vi "Filter Only Tomestones.vi"(8 "Error In":errorcluster, 11 "VI Bookmarks":T1[](array[typedef])) -> (0 "Error Out":errorcluster, 3 "Graves":T1[](array[typedef]))   [LabVIEW 2017, in "Graveyard.lvlib"]
doc: "Filters out all bookmarks that are NOT graves"
uses:
  Graveyard.lvlib
  VI Bookmark.ctl
  VI Information.ctl
  Application Information.ctl
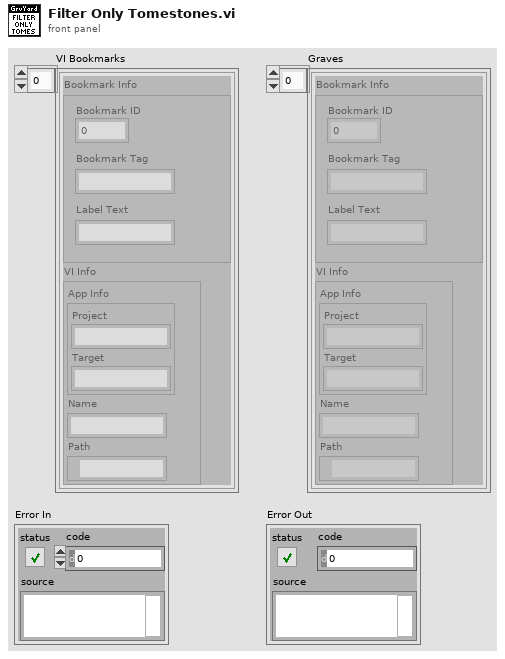
[diagram p1: front panel]
types:
  T1 = typedef "Graveyard.lvlib/VI Bookmark.ctl" = cluster{"Bookmark Info":cluster{"Bookmark ID":u32, "Bookmark Tag":string, "Label Text":string}, "VI Info":T2}
  T2 = typedef "Graveyard.lvlib/VI Information.ctl" = cluster{"App Info":T3, "Name":string, "Path":path}
  T3 = typedef "Graveyard.lvlib/Application Information.ctl" = cluster{"Project":string, "Target":string}
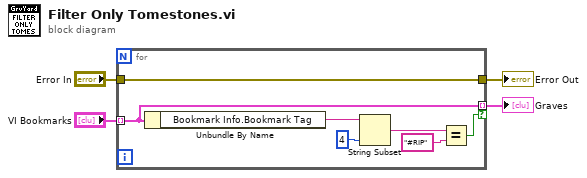
[diagram p0: block diagram]
diagram:
  n1 = for {
    tunnel: [w5] -> w1 mode=indexing if=w7
    tunnel: "Error In" -> [w8]
    tunnel: [w8] -> w3
    tunnel: "VI Bookmarks" -> [w5] mode=indexing
    n2 = Unbundle By Name(w5) -> ("Bookmark Info.Bookmark Tag"=w6:string)
    n3 = String Subset(string=w6, length (rest)=4 ("length (rest)")) -> (substring=w10:string)  [unwired: 1 in]
    n4 = Equal?(x=w10, y="#RIP") -> (x = y?=w7:bool)
  }
  "Error Out" <- w3
  "Graves" <- w1
